vi "S3DK GUI.vi"(8 "error in (no error)":errorcluster) -> (0 "error out":errorcluster)   [LabVIEW 2013, in "PMU Recorder Light.lvlib"]
uses:
  PMU Recorder Light.lvlib
  Phasor Data Concentrator Class/Phasor Data Concentrator.lvclass
  <vilib>/Utility/sysdir.llb/System Directory Type.ctl
  <vilib>/platform/TimedLoop/XDataNode/XDataNode.xnode
  <vilib>/Platform/TimedLoop/XDataNode/nitl_modes.ctl
  <vilib>/Platform/TimedLoop/XDataNode/XDNodeRunTimeDep.lvlib
  <vilib>/Platform/TimedLoop/XDataNode/wakeup.ctl
  <vilib>/Platform/TimedLoop/XDataNode/timing_clust.ctl
  Configuration Settings.ctl
  Setting Choice.ctl
panel:
  out "Number of bad dt":u64
  out "Latest Time Stamp":timestamp format="%<%X  %x>T"
  in  "Channel Selector":bool
  out "Manual Control":bool
  out "PDC Initialized":bool
  out "Queue Active":bool
  out "Connected":bool
  out "Configuration File Read":bool
  out "PDC Connected":bool
  out "Shutdown":bool
  out "Autostart":bool
  out "Bad Data Removal":bool
  out "Buffer Active":bool
  out "Configuration File Timeout":bool
  out "Configuration File Received":bool
  out "Initializing...":bool
  out "Bad Data?":bool
  out "Complex Bad":dbl(knob) scale=0.0..50.0
  out "Writing To File Buffer?":bool
  out "Lost File Buffer Data?":bool
  out "Writer Activity":dbl(knob) scale=0.0..100.0
  out "Buffer Queued?":bool
  out "Reader Activity":dbl(knob) scale=0.0..100.0
  out "Data?":bool
  out "Bad dt?":bool
  in  "Raw Data Panel":bool
  out "Worker Status":bool
  out "Secretary Pulse":bool
  out "Quitting...":bool
  out "Status":string="off"
  out "Data Rate":sgl=nan format="%#_6f"
  out "Control":enum32{"Auto", "Manual"}(tab)
  in  "Config":bool
  in  "Restart":bool
  in  "Quit":bool
  in  "Shutdown Logging":bool
  in  "Pause":bool
  in  "Startup":bool
  in  "Abort Wait":bool
  in  "PDC Initialize":bool
  in  "DLL Start Readers":bool
  in  "DLL Shutdown":bool
  in  "DLL Read Config":bool
  in  "DLL Wait for config":bool
  in  "DLL Initialize":bool
  in  "Quit 2":bool
  in  "Restart 2":bool
  in  "Config 2":bool
  in  "dt min":dbl=nan
  in  "dt max":dbl=nan
  in  "PRL Configuration":T1={"Connection Settings"={"IP-address"="127.0.0.1", "Port"="5001", "ID Code"=1001}, "Autostart"=FALSE, "Bad Data Removal"=TRUE, "Access Buffer Active"=TRUE, "Wait for Config Total Time [ms]"=2000, "Seconds to Wait if Config Fails [s]"=10, "Live Data Buffer Size"=5, "Number of Live Buffers in Access Buffer"=0, "Data Rate History"=100, "Complex Data Points Allowed Equal"=10, "Analog Data Points Allowed Equal"=50, "Number of Connection Attempts"=0, "Access Queue Active"=FALSE, "Access Buffer Size [hh:mm]"=600.0, "Sampling rate [Hz]"=nan, "Manual Control"=FALSE, "dt Tolerance [microseconds]"=10.0, "Wait for Config Timeout [ms]"=20, "Max Time Stamp Age Before Reconnect [s]"=10.0, "Poll New Data Timeout [ms]"=5} {"Access Buffer Size [hh:mm]" format="%<%H:%M>t"}
  # "INPUT"
  # "OUTPUT"
  # "INTERMEDIATE"
  # "v1.2  2013-08-01"
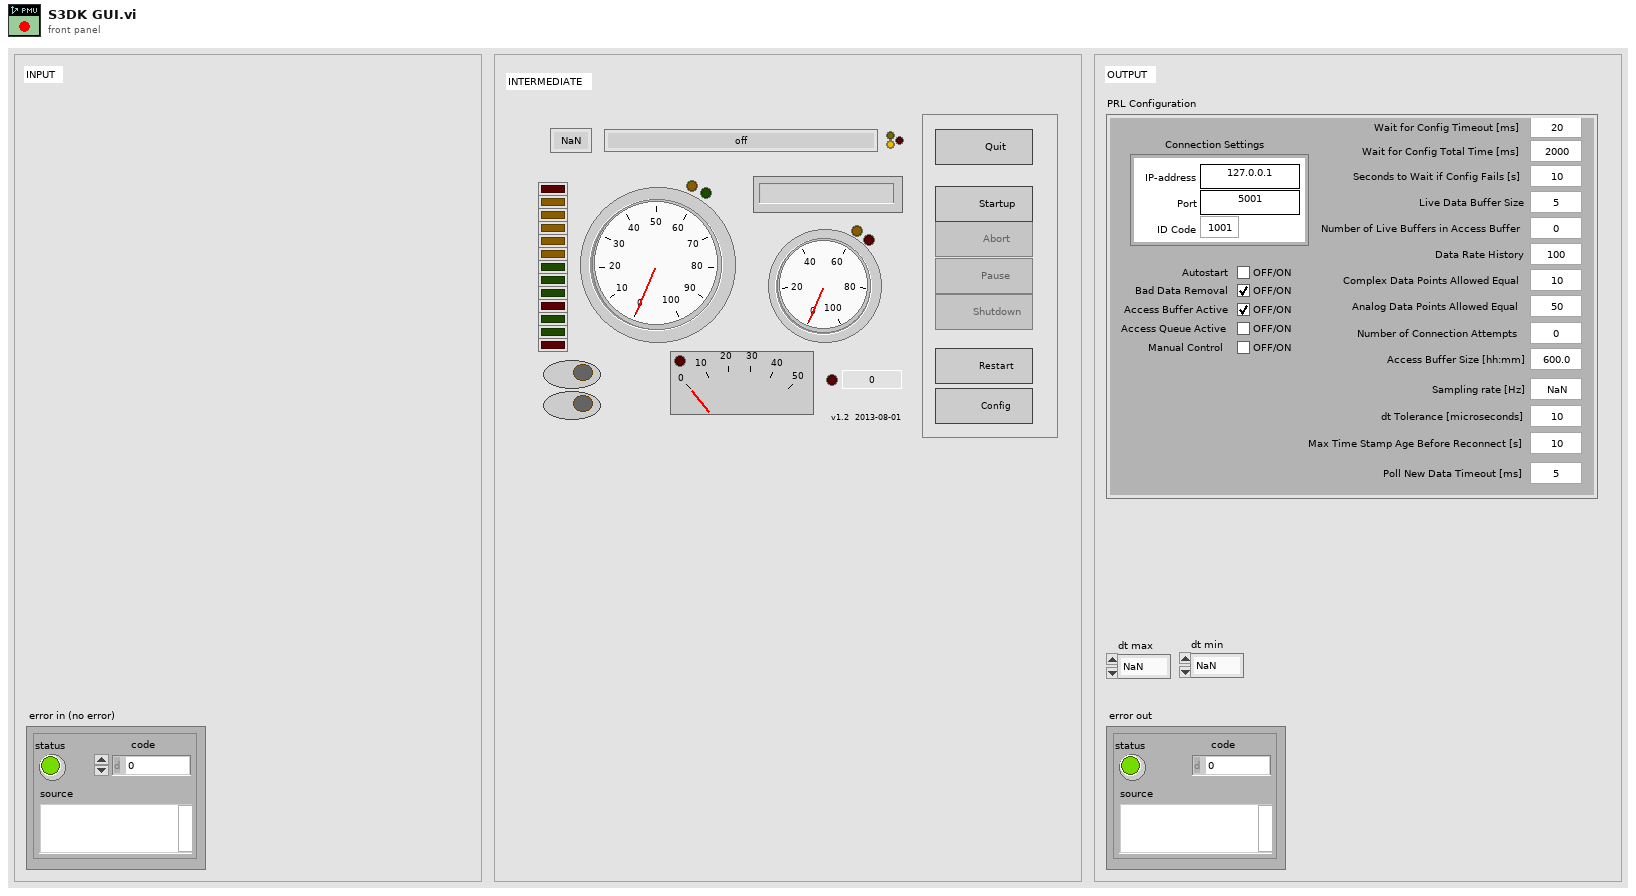
[diagram p1: front panel]
types:
  T1 = cluster{"Connection Settings":cluster{"IP-address":string, "Port":string, "ID Code":u32}, "Autostart":bool, "Bad Data Removal":bool, "Access Buffer Active":bool, "Wait for Config Total Time [ms]":i32, "Seconds to Wait if Config Fails [s]":i32, "Live Data Buffer Size":i32, "Number of Live Buffers in Access Buffer":i32, "Data Rate History":i32, "Complex Data Points Allowed Equal":i32, "Analog Data Points Allowed Equal":i32, "Number of Connection Attempts":i32, "Access Queue Active":bool, "Access Buffer Size [hh:mm]":dbl, "Sampling rate [Hz]":dbl, "Manual Control":bool, "dt Tolerance [microseconds]":dbl, "Wait for Config Timeout [ms]":i32, "Max Time Stamp Age Before Reconnect [s]":dbl, "Poll New Data Timeout [ms]":u16}
  T2 = typedef "PMU Recorder Light.lvlib/Setting Choice.ctl" = enum16{"Analog Data Points Allowed Equals", "Complex Data Points Allowed Equals", "Seconds Before Reset After Wait for Config Fails", "Number of Live Buffer in Access Buffer ", "Number of Connection Attempts", "Live Data Buffer Size", "dt Tolerance", "Data Rate History", "ALL"}
  T3 = typedef "PMU Recorder Light.lvlib/Configuration Settings.ctl" = cluster{"PRL Analog Data Points Allowed Equal":i32, "PRL Complex Data Points Allowed Equal":i32, "PRL Seconds Before Reset After Wait for Config Fails":i32, "PRL Number of Live Buffer in Access Buffer":i32, "PRL Number of Connection Attempts":i32, "PRL Live Data Buffer Size":i32, "PRL dt Tolerance":dbl, "PRL Data Rate History":i32}
  T4 = typedef "XDNodeRunTimeDep.lvlib/timing_clust.ctl" = cluster{"Expected End [f-1]":u64, "Actual End [f-1]":u64, "Finished Late? [f-1]":bool, "Expected End [i-1]":u64, "Actual End [i-1]":u64, "Finished Late? [i-1]":bool, "Expected Start [i]":u64, "Actual Start [i]":u64, "Expected Start [f]":u64, "Actual Start [f]":u64, "Source Name":string, "Structure Name":string, "Period":i64, "Deadline":i64, "Offset":i64, "Start":i64, "Priority":i32, "Timeout":i32, "Mode":T5, "Wakeup Reason":T6, "Error":errorcluster, "Source Type":string, "Secondary Source Type":string, "Global End Time":u64, "Global Start Time":u64, "Frame Duration":u64, "Iteration Duration":u64, "Assigned CPU":i32, "I/O Scan Engine Mode":u32}
  T5 = typedef "XDNodeRunTimeDep.lvlib/nitl_modes.ctl" = enum32{"No Change", "Process missed periods, maintain original phase", "Discard missed periods, maintain original phase", "Process missed periods, ignore original phase", "Discard missed periods, ignore original phase"}
  T6 = typedef "XDNodeRunTimeDep.lvlib/wakeup.ctl" = enum32{"Normal", "Aborted", "Asynchronous wakeup", "Timing source error", "Timed loop error", "Timeout"}
  T7 = enum8{"Enabled", "Disabled", "Disabled and Grayed Out"}
  T8 = typedef "System Directory Type.ctl" = i32
  T9 = cluster{"IP-address":string, "Port":string, "ID Code":u32}
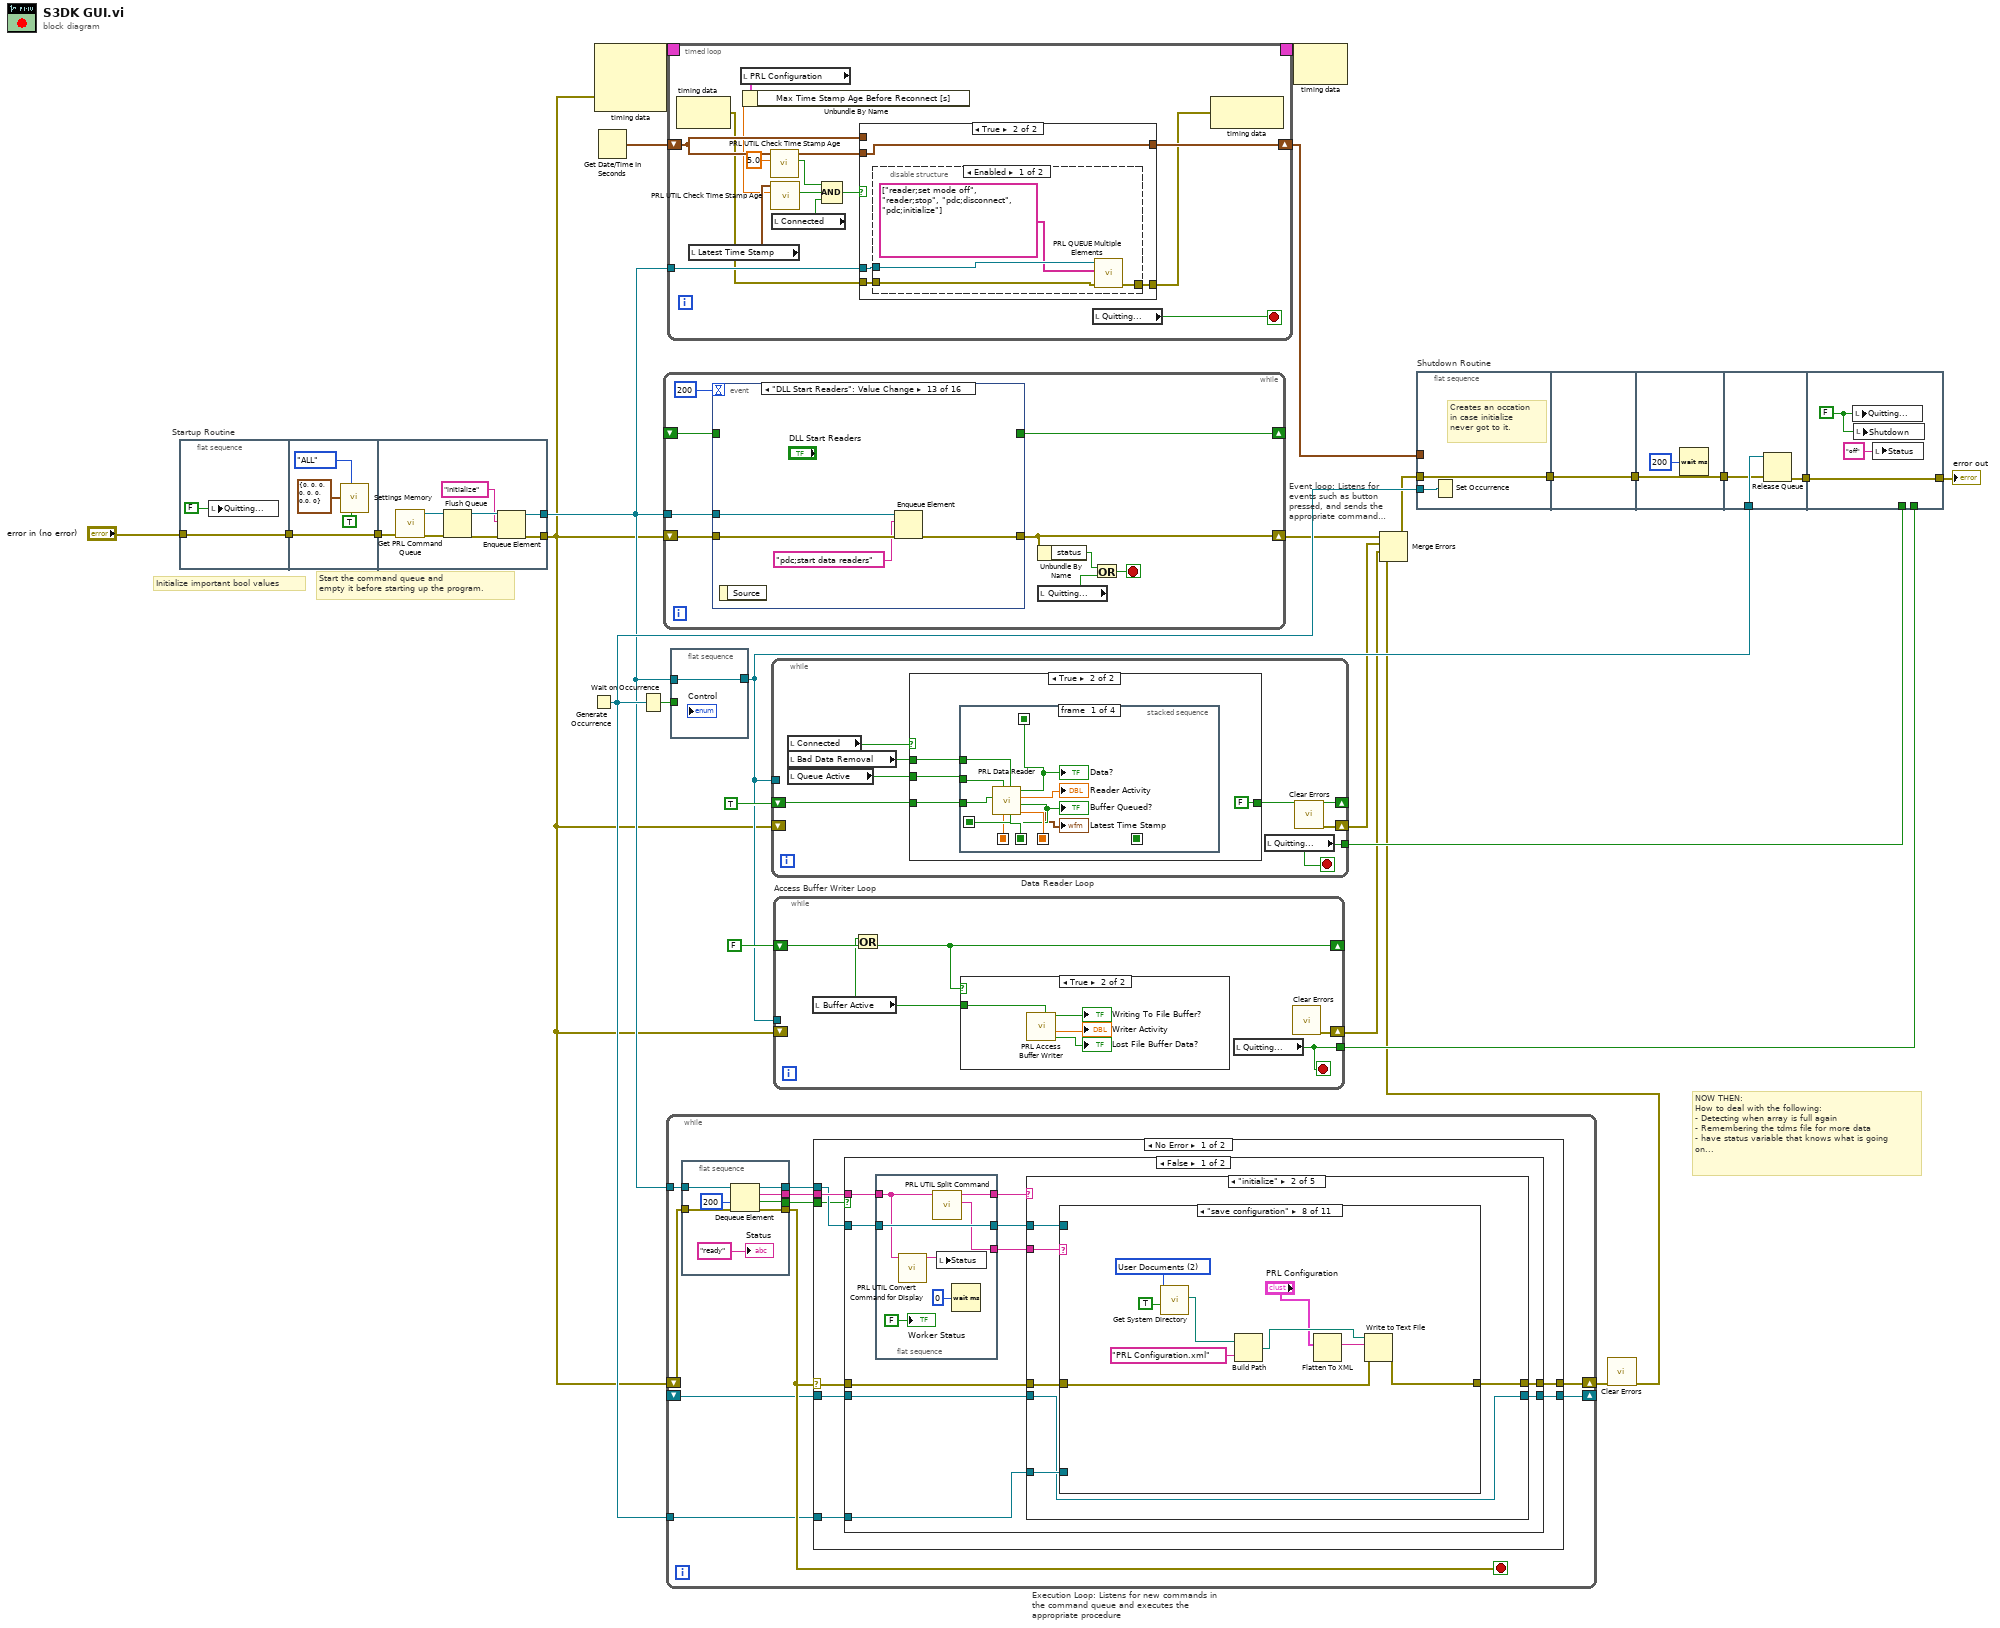
[diagram p0: block diagram]
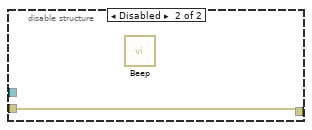
[diagram p3: hidden frame]
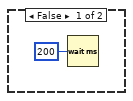
[diagram p4: hidden frame]
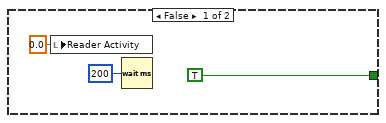
[diagram p5: hidden frame]
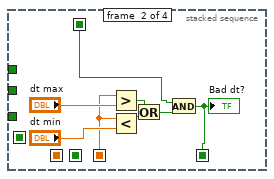
[diagram p6: hidden frame]
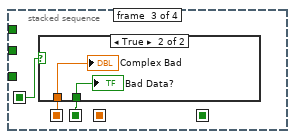
[diagram p7: hidden frame]
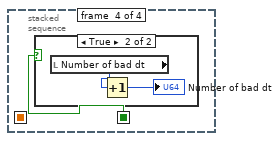
[diagram p9: hidden frame]
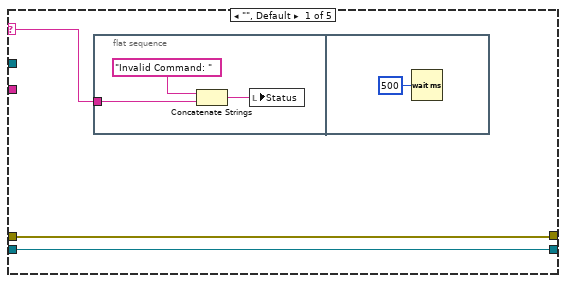
[diagram p11: hidden frame]
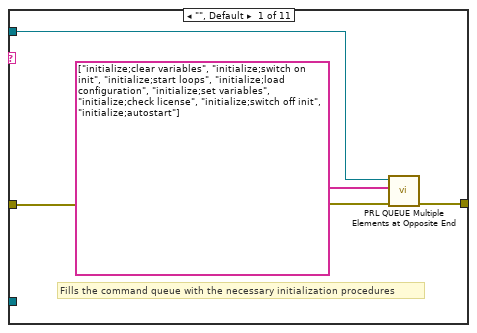
[diagram p12: hidden frame]
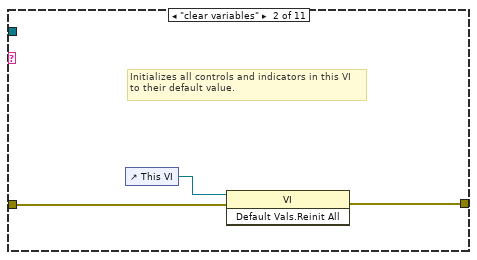
[diagram p13: hidden frame]
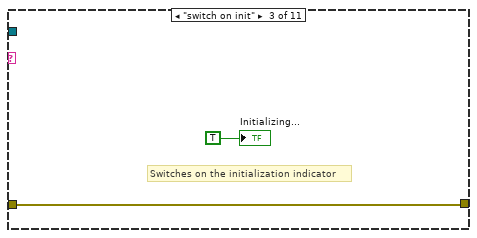
[diagram p14: hidden frame]
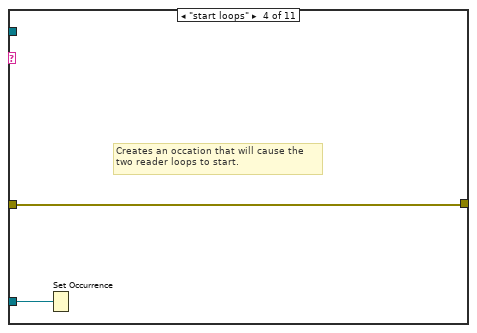
[diagram p15: hidden frame]
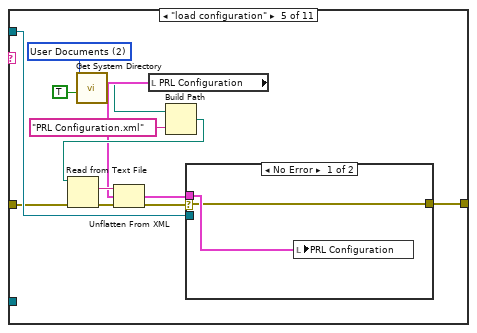
[diagram p16: hidden frame]
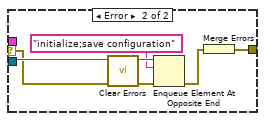
[diagram p17: hidden frame]
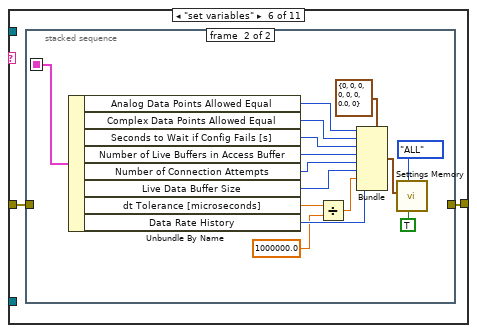
[diagram p18: hidden frame]
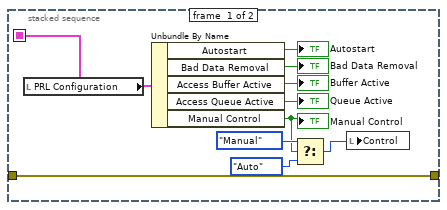
[diagram p19: hidden frame]
diagram:
  # "Initialize important bool values"
  # "Start the command queue and \nempty it before starting up the program."
  # "NOW THEN:\nHow to deal with the following:\n- Detecting when array is full again\n- Remembering the tdms file for more data\n- have status variable that knows what is going\non..."
  n1 = flat-sequence "Startup Routine" {
    tunnel: [w28] -> w2
    tunnel: "error in (no error)" -> [w28]
    tunnel: w2 -> [w33]
    tunnel: [w33] -> w1
    tunnel: [w39] -> w12
    tunnel: [w37] -> w18
    tunnel: w1 -> [w34]
    frame #0 {
      n2 = local write "Quitting..."(FALSE ("Exit?")) -> ()
    }
    frame #1 {
      n3 = call "Settings Memory.vi"("Write?"=TRUE, "Setting Choice"=Setting_Choice."ALL", "Input"=T3 {"PRL Analog Data Points Allowed Equal"=0, "PRL Complex Data Points Allowed Equal"=0, "PRL Seconds Before Reset After Wait for Config Fails"=0, "PRL Number of Live Buffer in Access Buffer"=0, "PRL Number of Connection Attempts"=0, "PRL Live Data Buffer Size"=0, "PRL dt Tolerance"=0.0, "PRL Data Rate History"=0} ("S3DK Config")) -> ()  [unwired: 6 in, 3 out]
    }
    frame #2 {
      n4 = call "Get PRL Command Queue.vi"("error in (no error)"=w34) -> ("error out"=w35:errorcluster, "PRL Command Queue"=w36:refnum<queue>)  [unwired: 9 in]
      n5 = Flush Queue(queue=w36, error in (no error)=w35) -> (queue out=w40:refnum<queue>, error out=w41:errorcluster)  [unwired: 1 out]
      n6 = Enqueue Element(queue=w40, element="initialize", error in (no error)=w41) -> (queue out=w37:refnum<queue>, error out=w39:errorcluster)  [unwired: 2 out]
    }
  }
  n7 = Generate Occurrence() -> (w24:refnum<k4>)
  n8 = node-c288(w12) -> (w20:T4)  [unwired: 2 in]
  n9 = Get Date/Time In Seconds() -> (seconds since 1Jan1904=w17:timestamp)
  n10 = Wait on Occurrence(2:w24) -> (0:w25:bool)  [unwired: 2 in]
  n11 = while "Event loop: Listens for events such as button pressed, and sends the appropriate commands to the\ncommand queue" {
    shift-right: [w45] -> w11
    shift-left: w12 -> [w46]
    tunnel: w18 -> [w47]
    shift-right: [w42] -> _
    shift-left: _ -> [w43]
    stop <- w49 stop-if-true
    n12 = event shown="[12] \"DLL Start Readers\": Value Change" {
      selector: _ -> [_ _ _ _ _ _ _ _ _ _ _ _ _ _ _ _]
      dyn-events: _ -> [_ _ _ _ _ _ _ _ _ _ _ _ _ _ _ _]
      timeout: 200 -> [_ _ _ _ _ _ _ _ _ _ _ _ _ _ _ _]
      tunnel: w47 -> [_ w58 w62 w66 w70 w74 w81 _ _ w107 w111 w115 w119 w123 w127 w131]
      tunnel: [w53 w56 w60 w63 w68 w71 w79 w82 w93 w105 w108 w112 w117 w120 w124 w129] -> w45
      tunnel: w46 -> [w53 w57 w61 w64 w69 w72 w80 w83 w94 w106 w109 w113 w118 w121 w125 w130]
      tunnel: w43 -> [w52 _ _ _ _ _ _ _ _ _ _ _ _ _ _ _]
      tunnel: [w51 _ _ _ _ _ _ _ _ _ _ _ _ _ _ _] -> w42
      event Timeout {
        n13 = event-data() -> ()  [unwired: 3 out]
        n14 = Not(x=w52) -> (.not. x?=w51:bool)
        "Secretary Pulse" <- w52
      }
      event "Quit", "Quit 2": Value Change {
        n15 = event-data() -> ()  [unwired: 2 out]
        n16 = Enqueue Element(queue=w58, element="shutdown", error in (no error)=w57) -> (error out=w56:errorcluster)  [unwired: 3 out]
        "Shutdown" <- TRUE ("Shutdown")
      }
      event "Restart", "Restart 2": Value Change {
        n17 = event-data() -> ()  [unwired: 2 out]
        n18 = Enqueue Element(queue=w62, element="initialize", error in (no error)=w61) -> (error out=w60:errorcluster)  [unwired: 3 out]
      }
      event "Startup": Value Change {
        n19 = event-data() -> ()  [unwired: 2 out]
        n20 = call "PRL QUEUE Multiple Elements.vi"("error in"=w64, "Elements to Add"=string[] ["pdc;initialize"], "queue"=w66) -> ("error out"=w63:errorcluster)  [unwired: 7 in, 1 out]
      }
      event "PDC Initialize": Value Change {
        n21 = event-data() -> ()  [unwired: 2 out]
        n22 = Enqueue Element(queue=w70, element="pdc;init", error in (no error)=w69) -> (error out=w68:errorcluster)  [unwired: 3 out]
      }
      event "Shutdown Logging": Value Change {
        n23 = event-data() -> ()  [unwired: 2 out]
        n24 = call "PRL QUEUE Multiple Elements.vi"("error in"=w72, "Elements to Add"=string[] ["reader;set mode off", "reader;stop", "pdc;disconnect"], "queue"=w74) -> ("error out"=w71:errorcluster)  [unwired: 7 in, 1 out]
      }
      event "Pause": Value Change {
        n25 = event-data() -> ()  [unwired: 2 out]
        n26 = Select(t=string[] ["reader;set mode paused", "reader;stop"] ("Elements to Add"), s="Pause", f=string[] ["reader;start", "reader;set mode logging"] ("Elements to Add")) -> (s? t:f=w76:string[])
        n27 = call "PRL QUEUE Multiple Elements.vi"("error in"=w80, "Elements to Add"=w76, "queue"=w81) -> ("error out"=w79:errorcluster)  [unwired: 7 in, 1 out]
      }
      event "Raw Data Panel": Value Change {
        n28 = event-data() -> ()  [unwired: 2 out]
        n29 = vi-ref "PRL Raw Data Viewer.vi"() -> (w85:refnum<vi>)
        n30 = case shown="True" "Raw Data Panel" {
          tunnel: w85 -> [w88 w92]
          tunnel: [w87 w90] -> w82
          tunnel: w83 -> [w86 w89]
          frame False {
            n31 = invoke class="VI" method="FP.Close"(reference=w88, error in=w86) -> (error out=w87:errorcluster)  [unwired: 1 in, 2 out]
          }
          frame True {
            n32 = invoke class="VI" method="FP.Open"(reference=w92, error in=w89, "Activate"=TRUE ("Activate?")) -> (error out=w90:errorcluster)  [unwired: 2 in, 4 out]
          }
        }
      }
      event "Channel Selector": Value Change {
        n33 = event-data() -> ()  [unwired: 2 out]
        n34 = vi-ref "PRL Channel Selector.vi"() -> (w96:refnum<vi>)
        n35 = case shown="False" "Channel Selector" {
          tunnel: w96 -> [w99 w103]
          tunnel: [w98 w101] -> w93
          tunnel: w94 -> [w97 w100]
          frame False {
            n36 = invoke class="VI" method="FP.Close"(reference=w99, error in=w97) -> (error out=w98:errorcluster)  [unwired: 1 in, 2 out]
          }
          frame True {
            n37 = invoke class="VI" method="FP.Open"(reference=w103, error in=w100, "Activate"=TRUE ("Activate?")) -> (error out=w101:errorcluster)  [unwired: 2 in, 4 out]
          }
        }
      }
      event "Config", "Config 2": Value Change {
        n38 = event-data() -> ()  [unwired: 2 out]
        n39 = Enqueue Element(queue=w107, element="initialize;configure", error in (no error)=w106) -> (error out=w105:errorcluster)  [unwired: 3 out]
      }
      event "DLL Initialize": Value Change {
        n40 = event-data() -> ()  [unwired: 2 out]
        n41 = Enqueue Element(queue=w111, element="pdc;dll initialize", error in (no error)=w109) -> (error out=w108:errorcluster)  [unwired: 3 out]
      }
      event "DLL Wait for config": Value Change {
        n42 = event-data() -> ()  [unwired: 2 out]
        n43 = Enqueue Element(queue=w115, element="pdc;dll wait for config", error in (no error)=w113) -> (error out=w112:errorcluster)  [unwired: 3 out]
      }
      event "DLL Start Readers": Value Change {
        n44 = event-data() -> ()  [unwired: 2 out]
        n45 = Enqueue Element(queue=w119, element="pdc;start data readers", error in (no error)=w118) -> (error out=w117:errorcluster)  [unwired: 3 out]
      }
      event "DLL Read Config": Value Change {
        n46 = event-data() -> ()  [unwired: 2 out]
        n47 = Enqueue Element(queue=w123, element="pdc;dll read config", error in (no error)=w121) -> (error out=w120:errorcluster)  [unwired: 3 out]
      }
      event "DLL Shutdown": Value Change {
        n48 = event-data() -> ()  [unwired: 2 out]
        n49 = Enqueue Element(queue=w127, element="pdc;disconnect", error in (no error)=w125) -> (error out=w124:errorcluster)  [unwired: 3 out]
      }
      event "Abort Wait": Value Change {
        n50 = event-data() -> ()  [unwired: 2 out]
        n51 = Enqueue Element(queue=w131, element="reader;set mode startup", error in (no error)=w130) -> (error out=w129:errorcluster)  [unwired: 3 out]
      }
    }
    n52 = Unbundle By Name(w45) -> ("status"=w50:bool)
    n53 = local read "Quitting..."() -> (w48:bool)
    n54 = Or(x=w50, y=w48) -> (x .or. y?=w49:bool)
  }
  n55 = while "Execution Loop: Listens for new commands in the command queue and executes the appropriate procedure" {
    tunnel: w18 -> [w141]
    tunnel: w24 -> [w136]
    shift-right: [w134] -> _
    shift-left: _ -> [w135]
    shift-right: [w132] -> w4
    shift-left: w12 -> [w133]
    stop <- w138 stop-if-true
    n56 = flat-sequence {
      tunnel: w141 -> [w149]
      tunnel: [w148] -> w140
      tunnel: [w147] -> w139
      tunnel: [w146] -> w138
      tunnel: [w143] -> w137
      tunnel: w133 -> [w142]
      frame #0 {
        n57 = Dequeue Element(queue=w149, timeout in ms (-1)=200, error in (no error)=w142) -> (queue out=w148:refnum<queue>, element=w147:string, timed out?=w143:bool, error out=w146:errorcluster)
        "Status" <- "ready" ("Status")
      }
    }
    n58 = case shown="No Error" w138 {
      selector: w138 -> [w151 w510]
      tunnel: w140 -> [w156 _]
      tunnel: w139 -> [w157 _]
      tunnel: w137 -> [w155 _]
      tunnel: w136 -> [w154 _]
      tunnel: w135 -> [w153 w511]
      tunnel: [w152 w511] -> w134
      tunnel: [w150 w510] -> w132
      frame No Error {
        n59 = case shown="False" w155 {
          tunnel: w157 -> [w167 _]
          tunnel: w156 -> [w166 _]
          tunnel: w154 -> [w162 _]
          tunnel: w153 -> [w161 w507]
          tunnel: [w160 w507] -> w152
          tunnel: w151 -> [w159 w506]
          tunnel: [w158 w506] -> w150
          frame False {
            n60 = flat-sequence {
              tunnel: [w503] -> w165
              tunnel: w167 -> [w501]
              tunnel: w166 -> [w505]
              tunnel: [w505] -> w164
              tunnel: [w502] -> w163
              frame #0 {
                n61 = call "PRL UTIL Convert Command for Display.vi"("Command In"=w501) -> ("Command Out"=w500:string)  [unwired: 10 in]
                n62 = call "PRL UTIL Split Command.vi"("Command"=w501) -> ("Parameters"=w502:string, "Command Out"=w503:string)  [unwired: 9 in]
                n63 = local write "Status"(w500) -> ()
                n64 = Wait (ms)(milliseconds to wait=u32 0) -> ()  [unwired: 1 out]
                "Worker Status" <- FALSE ("System Ready")
              }
            }
            n65 = case shown="\"initialize\"" w165 {
              selector: w165 -> [w170 _ _ _ _]
              tunnel: w164 -> [_ w180 w276 w429 w490]
              tunnel: w163 -> [_ w179 w277 w430 w489]
              tunnel: w162 -> [_ w178 _ _ _]
              tunnel: w161 -> [w169 w177 w275 w428 w488]
              tunnel: [w169 w177 w274 w428 w488] -> w160
              tunnel: w159 -> [w168 w176 w273 w427 w487]
              tunnel: [w168 w175 w272 w426 w486] -> w158
              frame "", Default {
                n66 = flat-sequence {
                  tunnel: w170 -> [w172]
                  frame #0 {
                    n67 = Concatenate Strings("Invalid Command: " ("Status"), w172) -> (w171:string)
                    n68 = local write "Status"(w171) -> ()
                  }
                  frame #1 {
                    n69 = Wait (ms)(milliseconds to wait=u32 500) -> ()  [unwired: 1 out]
                  }
                }
              }
              frame "initialize" {
                n70 = case shown="\"save configuration\"" w179 {
                  tunnel: w180 -> [w184 _ _ _ w198 _ _ _ _ w261 w265]
                  tunnel: w178 -> [_ _ _ w191 _ _ _ _ _ _ _]
                  tunnel: w176 -> [w182 w186 w188 w190 w193 w214 w240 w248 w256 w259 w267]
                  tunnel: [w181 w185 w188 w190 w192 w213 w241 w247 w256 w258 w268] -> w175
                  frame "", Default {
                    # "Fills the command queue with the necessary initialization procedures"
                    n71 = call "PRL QUEUE Multiple Elements at Opposite End.vi"("error in"=w182, "Elements to Add"=string[] ["initialize;clear variables", "initialize;switch on init", "initialize;start loops", "initialize;load configuration", "initialize;set variables", "initialize;check license", "initialize;switch off init", "initialize;autostart"], "queue"=w184) -> ("error out"=w181:errorcluster)  [unwired: 7 in, 1 out]
                  }
                  frame "clear variables" {
                    # "Initializes all controls and indicators in this VI\nto their default value."
                    n72 = control-ref of="This VI"() -> (w187:refnum<vi>)
                    n73 = invoke class="VI" method="Default Vals.Reinit All"(reference=w187, error in=w186) -> (error out=w185:errorcluster)  [unwired: 1 in, 2 out]
                  }
                  frame "switch on init" {
                    # "Switches on the initialization indicator"
                    "Initializing..." <- TRUE ("Initializing...")
                  }
                  frame "start loops" {
                    # "Creates an occation that will cause the \ntwo reader loops to start."
                    n74 = Set Occurrence(w191) -> ()
                  }
                  frame "load configuration" {
                    w196 = T8 2 items=["User Home"=0, "User Desktop"=1, "User Documents"=2, "User Application Data"=3, "User Preferences"=4, "User Temporary"=5, "Public Documents"=6, "Public Application Data"=7, "Public Preferences"=8, "Public Cache"=13, "System Core Libraries"=9, "System Installed Libraries"=10, "Application Files"=11, "Boot Volume Root"=12] ("system directory type")
                    n75 = call <vilib>:"Get System Directory.vi"("create directory if not found? (F)"=TRUE, "system directory type"=w196) -> ("system directory"=w194:path)  [unwired: 9 in]
                    n76 = local read "PRL Configuration"() -> (w200:T1)
                    n77 = Build Path(base path=w194, name or relative path="PRL Configuration.xml") -> (appended path=w201:path)
                    n78 = Read from Text File(file (use dialog)=w201, error in=w193) -> (text=w204:string, error out=w203:errorcluster)  [unwired: 2 in, 2 out]
                    n79 = Unflatten From XML(xml string=w204, type=w200, error in (no error)=w203) -> (value=w197:T1, error out=w199:errorcluster)
                    n80 = case shown="No Error" w199 {
                      selector: w199 -> [w205 w209]
                      tunnel: w198 -> [_ w212]
                      tunnel: w197 -> [w206 _]
                      tunnel: [w205 w207] -> w192
                      frame No Error {
                        n81 = local write "PRL Configuration"(w206) -> ()
                      }
                      frame Error {
                        n82 = call <vilib>:"Clear Errors.vi"("error in (no error)"=w209) -> ("error out"=w210:errorcluster)  [unwired: 5 in, 1 out]
                        n83 = Enqueue Element At Opposite End(queue=w212, element="initialize;save configuration", error in (no error)=w210) -> (error out=w208:errorcluster)  [unwired: 1 in, 2 out]
                        n84 = Merge Errors(w208) -> (w207:errorcluster)
                      }
                    }
                  }
                  frame "set variables" {
                    n85 = stacked-sequence {
                      seq-local: [w221 _] -> [_ w239]
                      tunnel: w214 -> [w215 _]
                      tunnel: [w215 _] -> w213
                      frame #0 {
                        n86 = local read "PRL Configuration"() -> (w221:T1)
                        n87 = Unbundle By Name(w221) -> ("Autostart"=→"Autostart":bool, "Bad Data Removal"=→"Bad Data Removal":bool, "Access Buffer Active"=→"Buffer Active":bool, "Access Queue Active"=→"Queue Active":bool, "Manual Control"=w216:bool)
                        "Manual Control" <- w216
                        n88 = Select(t=enum32{"Auto", "Manual"}."Manual" ("Control"), s=w216, f=enum32{"Auto", "Manual"}."Auto" ("Control")) -> (s? t:f=w219:enum32{"Auto", "Manual"})
                        n89 = local write "Control"(w219) -> ()
                      }
                      frame #1 {
                        n90 = Unbundle By Name(w239) -> ("Analog Data Points Allowed Equal"=w234:i32, "Complex Data Points Allowed Equal"=w233:i32, "Seconds to Wait if Config Fails [s]"=w232:i32, "Number of Live Buffers in Access Buffer"=w231:i32, "Number of Connection Attempts"=w230:i32, "Live Data Buffer Size"=w229:i32, "dt Tolerance [microseconds]"=w227:dbl, "Data Rate History"=w228:i32)
                        n91 = Divide(x=w227, y=1000000.0) -> (x/y=w225:dbl)
                        n92 = Bundle(cluster=T3 {"PRL Analog Data Points Allowed Equal"=0, "PRL Complex Data Points Allowed Equal"=0, "PRL Seconds Before Reset After Wait for Config Fails"=0, "PRL Number of Live Buffer in Access Buffer"=0, "PRL Number of Connection Attempts"=0, "PRL Live Data Buffer Size"=0, "PRL dt Tolerance"=0.0, "PRL Data Rate History"=0} ("S3DK Config"), "PRL Analog Data Points Allowed Equal"=w234, "PRL Complex Data Points Allowed Equal"=w233, "PRL Seconds Before Reset After Wait for Config Fails"=w232, "PRL Number of Live Buffer in Access Buffer"=w231, "PRL Number of Connection Attempts"=w230, "PRL Live Data Buffer Size"=w229, "PRL dt Tolerance"=w225, "PRL Data Rate History"=w228) -> (w235:T3)
                        n93 = call "Settings Memory.vi"("Write?"=TRUE, "Setting Choice"=Setting_Choice."ALL", "Input"=w235) -> ()  [unwired: 6 in, 3 out]
                      }
                    }
                  }
                  frame "check license" {
                    n94 = disable-structure shown="Enabled" {
                      disable-tunnel: [_ w246] -> w241
                      disable-tunnel: w240 -> [_ w246]
                      frame Disabled {
                        n95 = Get Date/Time In Seconds() -> (seconds since 1Jan1904=w244:timestamp)
                        n96 = Greater Or Equal?(x=w244, y=timestamp(3471375600 s since 1904-01-01)) -> (x >= y?=w242:bool)
                        n97 = case shown="True" w242 {
                          frame False {
                          }
                          frame True {
                            n98 = One Button Dialog(message="This version of the software \nis not licensed for use after \nJanuary 1st 2014.\n\nPlease contact Statnett R&D\nfor an upgrade.") -> ()  [unwired: 1 in, 1 out]
                          }
                        }
                      }
                      frame Enabled {
                        # "No License Check"
                      }
                    }
                  }
                  frame "save configuration" {
                    w251 = T8 2 items=["User Home"=0, "User Desktop"=1, "User Documents"=2, "User Application Data"=3, "User Preferences"=4, "User Temporary"=5, "Public Documents"=6, "Public Application Data"=7, "Public Preferences"=8, "Public Cache"=13, "System Core Libraries"=9, "System Installed Libraries"=10, "Application Files"=11, "Boot Volume Root"=12] ("system directory type")
                    n99 = call <vilib>:"Get System Directory.vi"("create directory if not found? (F)"=TRUE, "system directory type"=w251) -> ("system directory"=w249:path)  [unwired: 9 in]
                    n100 = Build Path(base path=w249, name or relative path="PRL Configuration.xml") -> (appended path=w253:path)
                    n101 = Flatten To XML(anything="PRL Configuration") -> (xml string=w254:string)
                    n102 = Write to Text File(file (use dialog)=w253, text=w254, error in=w248) -> (error out=w247:errorcluster)  [unwired: 1 in, 2 out]
                  }
                  frame "switch off init" {
                    n103 = local write "Initializing..."(FALSE ("Init")) -> ()
                  }
                  frame "autostart" {
                    n104 = local read "Autostart"() -> (w262:bool)
                    n105 = Select(t=string[] ["pdc;initialize"] ("Elements to Add"), s=w262, f=string[] ["reader;set mode off"] ("Elements to Add")) -> (s? t:f=w260:string[])
                    n106 = call "PRL QUEUE Multiple Elements.vi"("error in"=w259, "Elements to Add"=w260, "queue"=w261) -> ("error out"=w258:errorcluster)  [unwired: 7 in, 1 out]
                  }
                  frame "configure" {
                    n107 = local read "PRL Configuration"() -> (w271:T1)
                    n108 = call "PRL Configuration.vi"("Error In"=w267, "Configuration In"=w271) -> ("Error Out"=w266:errorcluster, "Configuration Out"=w270:T1)  [unwired: 8 in]
                    n109 = local write "PRL Configuration"(w270) -> ()
                    n110 = call "PRL QUEUE Multiple Elements at Opposite End.vi"("error in"=w266, "Elements to Add"=string[] ["initialize;save configuration", "initialize;set variables"], "queue"=w265) -> ("error out"=w268:errorcluster)  [unwired: 7 in, 1 out]
                  }
                }
              }
              frame "pdc" {
                n111 = case shown="\"read config\"" w277 {
                  tunnel: w276 -> [w282 _ w306 w327 w343 w365 w395 _ _ _]
                  tunnel: w275 -> [w280 _ w304 w326 w351 w372 w396 w400 w404 w410]
                  tunnel: [w280 w289 w296 w326 w345 w366 w392 w399 w403 w409] -> w274
                  tunnel: w273 -> [w279 w284 w298 w321 w342 w362 w386 w398 w402 w408]
                  tunnel: [w278 w283 w294 w320 w340 w360 w384 w397 w401 w407] -> w272
                  frame "initialize", Default {
                    n112 = call "PRL QUEUE Multiple Elements at Opposite End.vi"("error in"=w279, "Elements to Add"=string[] ["reader;set mode startup", "pdc;init object", "pdc;connect"], "queue"=w282) -> ("error out"=w278:errorcluster)  [unwired: 7 in, 1 out]
                  }
                  frame "init object" {
                    n113 = local read "PRL Configuration"() -> (w292:T1)
                    n114 = Unbundle By Name(w292) -> ("Connection Settings"=w291:T9, "Wait for Config Timeout [ms]"=w290:i32, "Wait for Config Total Time [ms]"=w286:i32)
                    n115 = control-ref of="Abort Wait"() -> (w285:refnum<vi>)
                    n116 = control-ref of="Quitting..."() -> (w287:refnum<vi>)
                    n117 = local write "Complex Bad"(0.0 ("Complex Bad")) -> ()
                    n118 = call "New.vi"("Abort Wait Reference 2"=w285, "Abort Wait Reference"=w287, "error in (no error)"=w284, "Wait for Config Total Time [ms]"=w286, "Wait for Config Timeout [ms]"=w290, "Connection Settings"=w291) -> ("error out"=w283:errorcluster, "Phasor Data Concentrator out"=w289:refnum<class "Phasor Data Concentrator.lvclass">)  [unwired: 4 in]
                    "PDC Initialized" <- TRUE ("PDC Initialized")
                  }
                  frame "connect" {
                    n119 = call "DLL Connect.vi"("error in (no error)"=w298, "Phasor Data Concentrator in"=w304) -> ("error out"=w303:errorcluster, "Phasor Data Concentrator out"=w305:refnum<class "Phasor Data Concentrator.lvclass">)  [unwired: 8 in]
                    n120 = call "DLL Get Status.vi"("error in (no error)"=w303, "Phasor Data Concentrator in"=w305) -> ("error out"=w297:errorcluster, "Configuration File Received"=→"Configuration File Received":bool, "Timeout"=→"Configuration File Timeout":bool, "Phasor Data Concentrator out"=w295:refnum<class "Phasor Data Concentrator.lvclass">, "Configuration Read OK"=→"Configuration File Read":bool, "PDC Connected"=w300:bool, "Data Rate"=→"Data Rate":sgl)  [unwired: 3 in]
                    "PDC Connected" <- w300
                    n121 = case shown="False" w300 {
                      tunnel: w306 -> [w311 w317]
                      tunnel: w297 -> [w309 w314]
                      tunnel: [w310 w315] -> w296
                      tunnel: w295 -> [w310 w315]
                      tunnel: [w308 w313] -> w294
                      frame False {
                        # "PDC Not Connected, so retrying"
                        n122 = call "PRL QUEUE Multiple Elements.vi"("error in"=w309, "Elements to Add"=string[] ["reader;set mode startup", "pdc;disconnect", "pdc;wait before reconnect"], "queue"=w311) -> ("error out"=w308:errorcluster)  [unwired: 7 in, 1 out]
                      }
                      frame True {
                        # "PDC Connected OK, so\nwaiting for config"
                        n123 = Enqueue Element(queue=w317, element="pdc;wait for config", error in (no error)=w314) -> (error out=w313:errorcluster)  [unwired: 3 out]
                      }
                    }
                  }
                  frame "wait before reconnect" {
                    n124 = call "Settings Memory.vi"("Setting Choice"=Setting_Choice."Seconds Before Reset After Wait for Config Fails") -> ("Output Int32"=w318:i32)  [unwired: 8 in, 2 out]
                    n125 = Tick Count (ms)() -> (millisecond timer value=w329:u32)
                    n126 = Multiply(x=w318, y=1000) -> (x*y=w328:i32)
                    n127 = while {
                      tunnel: w329 -> [w337]
                      tunnel: w328 -> [w335]
                      tunnel: [w333] -> w325
                      stop <- w334 stop-if-true
                      n128 = Tick Count (ms)() -> (millisecond timer value=w338:u32)
                      n129 = local read "Shutdown"() -> (w332:bool)
                      n130 = local read "Abort Wait"() -> (w331:bool)
                      n131 = Subtract(x=w338, y=w337) -> (x-y=w336:u32)
                      n132 = Greater?(x=w336, y=w335) -> (0:w333:bool)
                      n133 = Wait (ms)(milliseconds to wait=u32 20) -> ()  [unwired: 1 out]
                      n134 = Compound Arithmetic op=OR(w333, w332, w331) -> (w334:bool)
                    }
                    n135 = Select(t=string[] ["pdc;initialize", "reader;set mode logging"] ("Elements to Add"), s=w325, f=string[] ["reader;set mode off"] ("Elements to Add")) -> (s? t:f=w322:string[])
                    n136 = call "PRL QUEUE Multiple Elements.vi"("error in"=w321, "Elements to Add"=w322, "queue"=w327) -> ("error out"=w320:errorcluster)  [unwired: 7 in, 1 out]
                  }
                  frame "wait for config" {
                    n137 = call "DLL Wait for Config.vi"("error in (no error)"=w342, "Phasor Data Concentrator in"=w351) -> ("error out"=w346:errorcluster, "Phasor Data Concentrator out"=w347:refnum<class "Phasor Data Concentrator.lvclass">)  [unwired: 8 in]
                    n138 = call "DLL Get Status.vi"("error in (no error)"=w346, "Phasor Data Concentrator in"=w347) -> ("error out"=w341:errorcluster, "Configuration File Received"=w344:bool, "Timeout"=w348:bool, "Phasor Data Concentrator out"=w345:refnum<class "Phasor Data Concentrator.lvclass">, "Configuration Read OK"=w349:bool, "PDC Connected"=w350:bool)  [unwired: 3 in, 1 out]
                    n139 = case shown="False" w344 {
                      tunnel: w343 -> [w354 w359]
                      tunnel: w341 -> [w353 w357]
                      tunnel: [w352 w356] -> w340
                      frame False {
                        # "Configuration not received, so retrying..."
                        n140 = call "PRL QUEUE Multiple Elements.vi"("error in"=w353, "Elements to Add"=string[] ["reader;set mode startup", "pdc;disconnect", "pdc;wait before reconnect"], "queue"=w354) -> ("error out"=w352:errorcluster)  [unwired: 7 in, 1 out]
                      }
                      frame True {
                        # "Configuration received OK,\nso reading config"
                        n141 = Enqueue Element(queue=w359, element="pdc;read config", error in (no error)=w357) -> (error out=w356:errorcluster)  [unwired: 3 out]
                      }
                    }
                    n142 = local write "PDC Connected"(w350) -> ()
                    n143 = local write "Configuration File Timeout"(w348) -> ()
                    n144 = local write "Configuration File Received"(w344) -> ()
                    n145 = local write "Configuration File Read"(w349) -> ()
                  }
                  frame "read config" {
                    n146 = call "DLL Read Config.vi"("error in (no error)"=w362, "Phasor Data Concentrator in"=w372) -> ("error out"=w367:errorcluster, "Phasor Data Concentrator out"=w368:refnum<class "Phasor Data Concentrator.lvclass">)  [unwired: 8 in]
                    n147 = call "DLL Get Status.vi"("error in (no error)"=w367, "Phasor Data Concentrator in"=w368) -> ("error out"=w361:errorcluster, "Configuration File Received"=w370:bool, "Timeout"=w369:bool, "Phasor Data Concentrator out"=w366:refnum<class "Phasor Data Concentrator.lvclass">, "Configuration Read OK"=w364:bool, "PDC Connected"=w371:bool, "Data Rate"=w363:sgl)  [unwired: 3 in]
                    n148 = case shown="False" w364 {
                      tunnel: w365 -> [w375 w383]
                      tunnel: w363 -> [_ w380]
                      tunnel: w361 -> [w374 w378]
                      tunnel: [w373 w377] -> w360
                      frame False {
                        # "Configuration not read, so retrying..."
                        n149 = call "PRL QUEUE Multiple Elements.vi"("error in"=w374, "Elements to Add"=string[] ["reader;set mode startup", "pdc;disconnect", "pdc;wait before reconnect"], "queue"=w375) -> ("error out"=w373:errorcluster)  [unwired: 7 in, 1 out]
                      }
                      frame True {
                        # "Configuration read OK,\nso initializing readers"
                        n150 = local read "PRL Configuration"() -> (w381:T1)
                        n151 = Bundle By Name(cluster=w381, "Sampling rate [Hz]"=w380) -> (w379:T1)
                        n152 = local write "PRL Configuration"(w379) -> ()
                        n153 = Enqueue Element(queue=w383, element="pdc;initialize data readers", error in (no error)=w378) -> (error out=w377:errorcluster)  [unwired: 3 out]
                      }
                    }
                    n154 = local write "Data Rate"(w363) -> ()
                    n155 = local write "PDC Connected"(w371) -> ()
                    n156 = local write "Configuration File Timeout"(w369) -> ()
                    n157 = local write "Configuration File Received"(w370) -> ()
                    n158 = local write "Configuration File Read"(w364) -> ()
                  }
                  frame "initialize data readers" {
                    # "Initialize\n- Access Buffer Writer\n- DLL readers with number of channels\n- Data Reader with number of channels\n- Data Selector with channel names\n- Poll data timeout (this has an impact on the\n  data rate indicator\n\nAfter all is initialized, the Data Reader Loop is started"
                    n159 = local read "PRL Configuration"() -> (w389:T1)
                    n160 = Unbundle By Name(w389) -> ("Poll New Data Timeout [ms]"=w388:u16)
                    n161 = call "PRL Access Buffer Writer.vi"("Initialize?"=TRUE) -> ()  [unwired: 7 in, 4 out]
                    n162 = To Long Integer(number=w388) -> (32bit integer=w387:i32)
                    n163 = call "Initialize DLL Readers.vi"("error in (no error)"=w386, "Poll Timeout [5 ms]"=w387, "Phasor Data Concentrator in"=w396) -> ("error out"=w390:errorcluster, "Phasor Data Concentrator out"=w391:refnum<class "Phasor Data Concentrator.lvclass">)  [unwired: 7 in]
                    n164 = call "Initialize Channel Selector.vi"("error in (no error)"=w390, "Phasor Data Concentrator in"=w391) -> ("error out"=w385:errorcluster, "Phasor Data Concentrator out"=w392:refnum<class "Phasor Data Concentrator.lvclass">)  [unwired: 8 in]
                    n165 = Enqueue Element(queue=w395, element="reader;start", error in (no error)=w385) -> (error out=w384:errorcluster)  [unwired: 1 in, 2 out]
                  }
                  frame "start data stream" {
                    n166 = call "PDC Start Data Stream.vi"("error in (no error)"=w398, "Phasor Data Concentrator in"=w400) -> ("error out"=w397:errorcluster, "Phasor Data Concentrator out"=w399:refnum<class "Phasor Data Concentrator.lvclass">)  [unwired: 8 in]
                  }
                  frame "stop data stream" {
                    n167 = call "PDC Stop Data Stream.vi"("error in (no error)"=w402, "Phasor Data Concentrator in"=w404) -> ("error out"=w401:errorcluster, "Phasor Data Concentrator out"=w403:refnum<class "Phasor Data Concentrator.lvclass">)  [unwired: 8 in]
                  }
                  frame "disconnect" {
                    n168 = flat-sequence {
                      tunnel: w410 -> [w415]
                      tunnel: [w414] -> w406
                      tunnel: w408 -> [w412]
                      tunnel: [w411] -> w405
                      tunnel: [w423] -> w409
                      tunnel: w406 -> [w423]
                      tunnel: [w422] -> w407
                      tunnel: w405 -> [w422]
                      frame #0 {
                        # "Don't shutdown the dll if it has\nnot been initialized (this causes\nthe dll to hang for a while)."
                        n169 = local read "PDC Initialized"() -> (w413:bool)
                        n170 = case shown="True" w413 {
                          tunnel: w415 -> [w417 w421]
                          tunnel: [w417 w420] -> w414
                          tunnel: w412 -> [w416 w419]
                          tunnel: [w416 w418] -> w411
                          frame False {
                          }
                          frame True {
                            n171 = call "DLL Disconnect.vi"("error in (no error)"=w419, "Phasor Data Concentrator in"=w421) -> ("error out"=w418:errorcluster, "Phasor Data Concentrator out"=w420:refnum<class "Phasor Data Concentrator.lvclass">)  [unwired: 8 in]
                          }
                        }
                      }
                      frame #1 {
                        w425 = FALSE ("PDC Initialized")
                        n172 = local write "PDC Initialized"(w425) -> ()
                        n173 = local write "PDC Connected"(w425) -> ()
                        n174 = local write "Configuration File Timeout"(w425) -> ()
                        n175 = local write "Configuration File Received"(w425) -> ()
                        n176 = local write "Configuration File Read"(w425) -> ()
                        n177 = local write "Data Rate"(sgl nan ("Data Rate")) -> ()
                      }
                    }
                  }
                }
              }
              frame "reader" {
                n178 = case shown="\"start\"" w430 {
                  tunnel: w429 -> [w434 w440 w446 _ _ _ _]
                  tunnel: w427 -> [w432 w437 w444 w457 w465 w470 w485]
                  tunnel: [w431 w435 w443 w450 w459 w471 w479] -> w426
                  frame "initialize", Default {
                    n179 = Enqueue Element At Opposite End(queue=w434, element="reader;start", error in (no error)=w432) -> (error out=w431:errorcluster)  [unwired: 1 in, 2 out]
                  }
                  frame "start" {
                    n180 = Enqueue Element At Opposite End(queue=w440, element="pdc;start data stream", error in (no error)=w437) -> (queue out=w438:refnum<queue>, error out=w436:errorcluster)  [unwired: 1 in, 1 out]
                    n181 = Enqueue Element(queue=w438, element="reader;set mode logging", error in (no error)=w436) -> (error out=w435:errorcluster)  [unwired: 3 out]
                    "Connected" <- TRUE ("Logging")
                  }
                  frame "stop" {
                    n182 = flat-sequence {
                      frame #0 {
                        n183 = local write "Connected"(FALSE ("Logging")) -> ()
                      }
                      frame #1 {
                        n184 = Wait (ms)(milliseconds to wait=u32 100) -> ()  [unwired: 1 out]
                      }
                    }
                    n185 = Enqueue Element At Opposite End(queue=w446, element="pdc;stop data stream", error in (no error)=w444) -> (error out=w443:errorcluster)  [unwired: 1 in, 2 out]
                  }
                  frame "set mode off" {
                    w449 = T7."Disabled and Grayed Out" ("Disabled")
                    w455 = T7."Enabled" ("Disabled")
                    n186 = property on="Startup" class="Bool"(error in=w457, "DisabledEnum"=w455) -> (error out=w456:errorcluster)  [unwired: 1 in, 1 out]
                    n187 = property on="Config" class="Bool"(error in=w456, "DisabledEnum"=w455) -> (error out=w454:errorcluster)  [unwired: 1 in, 1 out]
                    n188 = property on="Restart" class="Bool"(error in=w454, "DisabledEnum"=w455) -> (error out=w453:errorcluster)  [unwired: 1 in, 1 out]
                    n189 = property on="Shutdown Logging" class="Bool"(error in=w453, "DisabledEnum"=w449) -> (error out=w452:errorcluster)  [unwired: 1 in, 1 out]
                    n190 = property on="Pause" class="Bool (strict)"(error in=w452, "DisabledEnum"=w449) -> (error out=w451:errorcluster)  [unwired: 1 in, 1 out]
                    n191 = property on="Abort Wait" class="Bool (strict)"(error in=w451, "DisabledEnum"=w449) -> (error out=w450:errorcluster)  [unwired: 1 in, 1 out]
                  }
                  frame "set mode startup" {
                    w458 = T7."Disabled and Grayed Out" ("Disabled")
                    n192 = property on="Abort Wait" class="Bool (strict)"(error in=w465, "DisabledEnum"=T7."Enabled" ("Disabled")) -> (error out=w464:errorcluster)  [unwired: 1 in, 1 out]
                    n193 = local write "Abort Wait"(FALSE ("Abort Wait")) -> ()
                    n194 = property on="Config" class="Bool"(error in=w464, "DisabledEnum"=w458) -> (error out=w463:errorcluster)  [unwired: 1 in, 1 out]
                    n195 = property on="Restart" class="Bool"(error in=w463, "DisabledEnum"=w458) -> (error out=w462:errorcluster)  [unwired: 1 in, 1 out]
                    n196 = property on="Shutdown Logging" class="Bool"(error in=w462, "DisabledEnum"=w458) -> (error out=w461:errorcluster)  [unwired: 1 in, 1 out]
                    n197 = property on="Pause" class="Bool (strict)"(error in=w461, "DisabledEnum"=w458) -> (error out=w460:errorcluster)  [unwired: 1 in, 1 out]
                    n198 = property on="Startup" class="Bool"(error in=w460, "DisabledEnum"=w458) -> (error out=w459:errorcluster)  [unwired: 1 in, 1 out]
                  }
                  frame "set mode logging" {
                    w468 = T7."Disabled and Grayed Out" ("Disabled")
                    w469 = T7."Enabled" ("Disabled")
                    n199 = property on="Pause" class="Bool (strict)"(error in=w470, "DisabledEnum"=w469) -> (error out=w476:errorcluster)  [unwired: 1 in, 1 out]
                    n200 = property on="Shutdown Logging" class="Bool"(error in=w476, "DisabledEnum"=w469) -> (error out=w475:errorcluster)  [unwired: 1 in, 1 out]
                    n201 = property on="Config" class="Bool"(error in=w475, "DisabledEnum"=w468) -> (error out=w474:errorcluster)  [unwired: 1 in, 1 out]
                    n202 = property on="Restart" class="Bool"(error in=w474, "DisabledEnum"=w468) -> (error out=w473:errorcluster)  [unwired: 1 in, 1 out]
                    n203 = property on="Abort Wait" class="Bool (strict)"(error in=w473, "DisabledEnum"=w468) -> (error out=w472:errorcluster)  [unwired: 1 in, 1 out]
                    n204 = property on="Startup" class="Bool"(error in=w472, "DisabledEnum"=w468) -> (error out=w471:errorcluster)  [unwired: 1 in, 1 out]
                  }
                  frame "set mode paused" {
                    w477 = T7."Disabled and Grayed Out" ("Disabled")
                    w483 = T7."Enabled" ("Disabled")
                    n205 = property on="Shutdown Logging" class="Bool"(error in=w485, "DisabledEnum"=w483) -> (error out=w484:errorcluster)  [unwired: 1 in, 1 out]
                    n206 = property on="Pause" class="Bool (strict)"(error in=w484, "DisabledEnum"=w483) -> (error out=w481:errorcluster)  [unwired: 1 in, 1 out]
                    n207 = property on="Config" class="Bool"(error in=w481, "DisabledEnum"=w477) -> (error out=w482:errorcluster)  [unwired: 1 in, 1 out]
                    n208 = property on="Restart" class="Bool"(error in=w482, "DisabledEnum"=w477) -> (error out=w478:errorcluster)  [unwired: 1 in, 1 out]
                    n209 = property on="Abort Wait" class="Bool (strict)"(error in=w478, "DisabledEnum"=w477) -> (error out=w480:errorcluster)  [unwired: 1 in, 1 out]
                    n210 = property on="Startup" class="Bool"(error in=w480, "DisabledEnum"=w477) -> (error out=w479:errorcluster)  [unwired: 1 in, 1 out]
                  }
                }
              }
              frame "shutdown" {
                n211 = case shown="\"quit\"" w489 {
                  tunnel: w490 -> [w494 _]
                  tunnel: w487 -> [w492 w498]
                  tunnel: [w491 w497] -> w486
                  frame "", Default {
                    n212 = local write "Shutdown"(TRUE ("Shutdown")) -> ()
                    n213 = call "PRL QUEUE Multiple Elements.vi"("error in"=w492, "Elements to Add"=string[] ["reader;stop", "reader;set mode off", "pdc;disconnect", "shutdown;quit"], "queue"=w494) -> ("error out"=w491:errorcluster)  [unwired: 7 in, 1 out]
                  }
                  frame "quit" {
                    w496 = TRUE ("Quitting...")
                    # "Make sure\nthis loop stops"
                    n214 = Bundle(cluster=w498, "status"=w496) -> (w497:errorcluster)  [unwired: 2 in]
                    "Quitting..." <- w496
                  }
                }
              }
            }
          }
          frame True {
            n215 = local write "Worker Status"(TRUE ("System Ready")) -> ()
            n216 = Wait (ms)(milliseconds to wait=u32 200) -> ()  [unwired: 1 out]
          }
        }
      }
      frame Error {
      }
    }
  }
  n217 = timed-loop {
    timing: w20 -> [_]
    timing-out: [_] -> w19
    shift-right: [w518] -> w16
    shift-left: w17 -> [w519]
    tunnel: w18 -> [w522]
    stop <- w521 stop-if-true
    n218 = node-c288() -> (w513:errorcluster)  [unwired: 1 in]
    n219 = local read "Latest Time Stamp"() -> (w526:timestamp)
    n220 = local read "PRL Configuration"() -> (w515:T1)
    n221 = Unbundle By Name(w515) -> ("Max Time Stamp Age Before Reconnect [s]"=w514:dbl)
    n222 = call "PRL UTIL Check Time Stamp Age.vi"("Max Age Allowed [s]"=5.0, "Time Stamp to Check"=w519) -> ("Trigger"=w525:bool, "Latest Time Stamp"=w520:timestamp)  [unwired: 8 in]
    n223 = call "PRL UTIL Check Time Stamp Age.vi"("Max Age Allowed [s]"=w514, "Time Stamp to Check"=w526) -> ("Trigger"=w524:bool)  [unwired: 8 in, 1 out]
    n224 = local read "Connected"() -> (w516:bool)
    n225 = Compound Arithmetic op=AND(w525, w524, w516) -> (w523:bool)
    n226 = case shown="True" w523 {
      tunnel: w522 -> [_ w532]
      tunnel: w520 -> [_ w531]
      tunnel: w519 -> [w528 _]
      tunnel: [w528 w531] -> w518
      tunnel: w513 -> [w527 w530]
      tunnel: [w527 w529] -> w512
      frame False {
      }
      frame True {
        n227 = disable-structure shown="Enabled" {
          disable-tunnel: w532 -> [w536 _]
          disable-tunnel: w530 -> [w534 w537]
          disable-tunnel: [w533 w537] -> w529
          frame Enabled {
            n228 = call "PRL QUEUE Multiple Elements.vi"("error in"=w534, "Elements to Add"=string[] ["reader;set mode off", "reader;stop", "pdc;disconnect", "pdc;initialize"], "queue"=w536) -> ("error out"=w533:errorcluster)  [unwired: 7 in, 1 out]
          }
          frame Disabled {
            n229 = call <vilib>:"Beep.vi"() -> ()  [unwired: 12 in]
          }
        }
      }
    }
    n230 = local read "Quitting..."() -> (w521:bool)
    n231 = node-c288(w512) -> ()  [unwired: 1 out]
  }
  n232 = flat-sequence {
    tunnel: w25 -> [_]
    tunnel: [w543] -> w21
    tunnel: w18 -> [w543]
    frame #0 {
    }
  }
  n233 = while "Data Reader Loop" {
    tunnel: w21 -> [_]
    tunnel: [w550] -> w27
    shift-right: [w548] -> _
    shift-left: TRUE ("Data?") -> [w549]
    shift-right: [w544] -> w10
    shift-left: w12 -> [_]
    stop <- w550 stop-if-true
    n234 = local read "Connected"() -> (w546:bool)
    n235 = local read "Bad Data Removal"() -> (w547:bool)
    n236 = local read "Queue Active"() -> (w545:bool)
    n237 = case shown="True" w546 {
      tunnel: w549 -> [_ w557]
      tunnel: [TRUE ("Data?") FALSE ("Data?")] -> w548
      tunnel: w547 -> [_ w555]
      tunnel: w545 -> [_ w554]
      frame False {
        n238 = local write "Reader Activity"(0.0 ("Data Rate")) -> ()
        n239 = Wait (ms)(milliseconds to wait=u32 200) -> ()  [unwired: 1 out]
      }
      frame True {
        n240 = stacked-sequence {
          seq-local: [w565 _ _ _] -> [_ w573 _ _]
          seq-local: [w564 _ _ _] -> [_ w571 _ _]
          seq-local: [w563 _ _ _] -> [_ _ w576 _]
          seq-local: [w562 _ _ _] -> [_ _ w578 _]
          seq-local: [w561 _ _ _] -> [_ _ w577 _]
          seq-local: [_ w568 _ _] -> [_ _ _ w581]
          tunnel: w557 -> [w566 _ _ _]
          tunnel: w555 -> [w560 _ _ _]
          tunnel: w554 -> [w559 _ _ _]
          frame #0 {
            n241 = call "PRL Data Reader.vi"("Remove Bad Data?"=w560, "Queue Active?"=w559, "Initialize Time"=w566) -> ("dt (ms)"=w565:dbl, "Buffer Queued?"=w562:bool, "Data Rate"=→"Reader Activity":dbl, "Data?"=w564:bool, "Bad Data?"=w563:bool, "Bad Data Ratio"=w561:dbl, "Latest Time Stamp"=→"Latest Time Stamp":timestamp)  [unwired: 2 in]
            "Data?" <- w564
            "Buffer Queued?" <- w562
          }
          frame #1 {
            n242 = Greater?(x=w573, y="dt max") -> (0:w570:bool)
            n243 = Less?(x=w573, y="dt min") -> (x < y?=w569:bool)
            n244 = Or(x=w570, y=w569) -> (x .or. y?=w572:bool)
            n245 = And(x=w571, y=w572) -> (x .and. y?=w568:bool)
            "Bad dt?" <- w568
          }
          frame #2 {
            n246 = case shown="True" w578 {
              tunnel: w577 -> [_ w580]
              tunnel: w576 -> [_ w579]
              frame False {
              }
              frame True {
                "Complex Bad" <- w580
                "Bad Data?" <- w579
              }
            }
          }
          frame #3 {
            n247 = case shown="True" w581 {
              frame False {
              }
              frame True {
                n248 = local read "Number of bad dt"() -> (w582:u64)
                n249 = Increment(x=w582) -> (x+1=→"Number of bad dt":u64)
              }
            }
          }
        }
      }
    }
    n250 = local read "Quitting..."() -> (w550:bool)
    n251 = call <vilib>:"Clear Errors.vi"() -> ("error out"=w544:errorcluster)  [unwired: 6 in, 1 out]
  }
  n252 = while "Access Buffer Writer Loop" {
    shift-right: [w586] -> _
    shift-left: FALSE ("Data?") -> [w588]
    tunnel: [w587] -> w22
    tunnel: w21 -> [_]
    shift-right: [w584] -> w9
    shift-left: w12 -> [_]
    stop <- w587 stop-if-true
    n253 = local read "Buffer Active"() -> (w585:bool)
    n254 = Or(x=w585, y=w588) -> (x .or. y?=w586:bool)
    n255 = case shown="True" w586 {
      tunnel: w585 -> [_ w593]
      frame False {
        n256 = Wait (ms)(milliseconds to wait=u32 200) -> ()  [unwired: 1 out]
      }
      frame True {
        n257 = call "PRL Access Buffer Writer.vi"("Write?"=w593) -> ("Lost Data?"=→"Lost File Buffer Data?":bool, "Activity Monitor"=→"Writer Activity":dbl, "Writing?"=→"Writing To File Buffer?":bool)  [unwired: 7 in, 1 out]
      }
    }
    n258 = local read "Quitting..."() -> (w587:bool)
    n259 = call <vilib>:"Clear Errors.vi"() -> ("error out"=w584:errorcluster)  [unwired: 6 in, 1 out]
  }
  n260 = node-c288(w19) -> ()  [unwired: 1 out]
  n261 = flat-sequence "Shutdown Routine" {
    tunnel: w24 -> [w595]
    tunnel: w16 -> [_]
    tunnel: w8 -> [w594]
    tunnel: [w594] -> w5
    tunnel: [w596] -> w6
    tunnel: w5 -> [w596]
    tunnel: [w597] -> w7
    tunnel: w6 -> [w597]
    tunnel: w21 -> [w601]
    tunnel: [w600] -> w13
    tunnel: w7 -> [w599]
    tunnel: w27 -> [_]
    tunnel: w22 -> [_]
    tunnel: [w602] -> w14
    tunnel: w13 -> [w602]
    frame #0 {
      # "Creates an occation\nin case initialize\nnever got to it."
      n262 = Set Occurrence(w595) -> ()
    }
    frame #1 {
    }
    frame #2 {
      n263 = Wait (ms)(milliseconds to wait=u32 200) -> ()  [unwired: 1 out]
    }
    frame #3 {
      n264 = Release Queue(queue=w601, error in (no error)=w599) -> (error out=w600:errorcluster)  [unwired: 3 out]
    }
    frame #4 {
      w604 = FALSE ("Exit?")
      n265 = local write "Quitting..."(w604) -> ()
      n266 = local write "Shutdown"(w604) -> ()
      n267 = local write "Status"("off" ("Status")) -> ()
    }
  }
  n268 = call <vilib>:"Clear Errors.vi"("error in (no error)"=w4) -> ("error out"=w3:errorcluster)  [unwired: 5 in, 1 out]
  n269 = Merge Errors(w11, w10, w9, w3) -> (w8:errorcluster)
  "error out" <- w14
